vi "Insert SubVI.vi"(11 "Sub UI":refnum<vi>[](array[refnum])) -> ()   [LabVIEW 2019]
uses:
  <vilib>/Utility/miscctls.llb/LVPositionTypeDef.ctl
panel:
  in  "TVertical/FHorizantal":bool
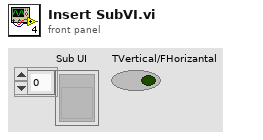
[diagram p1: front panel]
types:
  T1 = typedef "LVPositionTypeDef.ctl" = cluster{"Left":i32, "Top":i32}
  T2 = typedef "LVPointTypeDef.ctl" = cluster{"Horizontal":i16, "Vertical":i16}
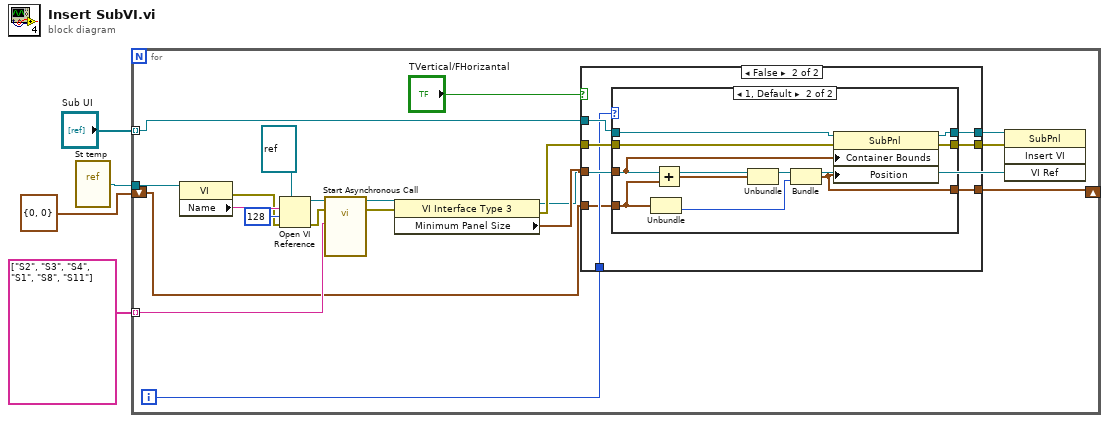
[diagram p0: block diagram]
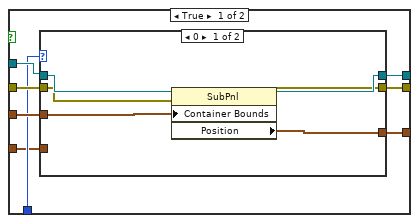
[diagram p2: hidden frame]
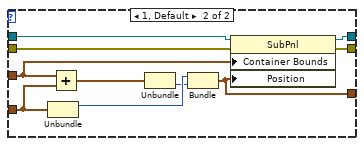
[diagram p3: hidden frame]
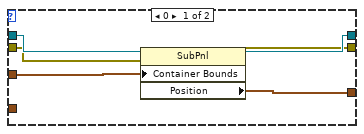
[diagram p4: hidden frame]
diagram:
  n1 = vi-ref "St temp.vi"() -> (w3:refnum<vi>)
  n2 = for {
    tunnel: "Sub UI" -> [w16] mode=indexing
    tunnel: w3 -> [w24]
    tunnel: string[] ["S2", "S3", "S4", "S1", "S8", "S11"] -> [w18] mode=indexing
    shift-right: [w7] -> _
    shift-left: T1 {"Left"=0, "Top"=0} ("Position") -> [w6]
    i -> [w8]
    n3 = property class="VI"(reference=w24) -> (error out=w20:errorcluster, "Name"=w23:string)  [unwired: 1 in, 1 out]
    n4 = Open VI Reference(type specifier VI Refnum (for type only)=refnum<vi> refnum, vi path=w23, options=128, error in (no error)=w20) -> (vi reference=w19:refnum<vi>, error out=w14:errorcluster)  [unwired: 2 in]
    n5 = call-by-ref "Start Asynchronous Call"(reference=w19, error in=w14, "Station Name"=w18) -> (reference out=w17:refnum<vi>, error out=w13:errorcluster)  [unwired: 11 in]
    n6 = property class="VI Interface Type 3"(reference=w17, error in=w13) -> (reference out=w9:refnum<vi>, error out=w12:errorcluster, "Minimum Panel Size"=w15:T2)
    n7 = case shown="False" "TVertical/FHorizantal" {
      tunnel: w16 -> [w32 w56]
      tunnel: w15 -> [w31 w55]
      tunnel: w12 -> [w30 w54]
      tunnel: [w29 w53] -> w11
      tunnel: [w28 w52] -> w10
      tunnel: w8 -> [w27 w51]
      tunnel: [w26 w50] -> w7
      tunnel: w6 -> [w25 w49]
      frame True {
        n8 = case shown="0" w27 {
          tunnel: w32 -> [w38 w48]
          tunnel: w31 -> [w36 w44]
          tunnel: w30 -> [w34 w47]
          tunnel: [w37 w46] -> w29
          tunnel: [w33 w45] -> w28
          tunnel: [w35 w39] -> w26
          tunnel: w25 -> [_ w43]
          frame 0 {
            n9 = property class="SubPnl"(reference=w38, error in=w34, "Container Bounds"=w36) -> (reference out=w37:refnum<vi>, error out=w33:errorcluster, "Position"=w35:T1)
          }
          frame 1, Default {
            n10 = Unbundle(w43) -> ("Left"=w41:i32)  [unwired: 1 out]
            n11 = Add(x=w44, y=w43) -> (x+y=w42:T1)
            n12 = Unbundle(w42) -> ("Top"=w40:i32)  [unwired: 1 out]
            n13 = Bundle("Left"=w41, "Top"=w40) -> (w39:cluster{"Left":i32, "Top":i32})  [unwired: 1 in]
            n14 = property class="SubPnl"(reference=w48, error in=w47, "Container Bounds"=w44, "Position"=w39) -> (reference out=w46:refnum<vi>, error out=w45:errorcluster)
          }
        }
      }
      frame False {
        n15 = case shown="1, Default" w51 {
          tunnel: w56 -> [w62 w72]
          tunnel: w55 -> [w60 w68]
          tunnel: w54 -> [w58 w71]
          tunnel: [w61 w70] -> w53
          tunnel: [w57 w69] -> w52
          tunnel: [w59 w65] -> w50
          tunnel: w49 -> [_ w67]
          frame 0 {
            n16 = property class="SubPnl"(reference=w62, error in=w58, "Container Bounds"=w60) -> (reference out=w61:refnum<vi>, error out=w57:errorcluster, "Position"=w59:T1)
          }
          frame 1, Default {
            n17 = Unbundle(w67) -> ("Top"=w63:i32)  [unwired: 1 out]
            n18 = Add(x=w68, y=w67) -> (x+y=w66:T1)
            n19 = Unbundle(w66) -> ("Left"=w64:i32)  [unwired: 1 out]
            n20 = Bundle("Left"=w64, "Top"=w63) -> (w65:cluster{"Left":i32, "Top":i32})  [unwired: 1 in]
            n21 = property class="SubPnl"(reference=w72, error in=w71, "Container Bounds"=w68, "Position"=w65) -> (reference out=w70:refnum<vi>, error out=w69:errorcluster)
          }
        }
      }
    }
    n22 = invoke class="SubPnl" method="Insert VI"(reference=w11, error in=w10, "VI Ref"=w9) -> ()  [unwired: 1 in, 4 out]
  }
